vi "Read ZY_control.vi"(8 "error in (no error)":errorcluster, 11 "reg in":refnum<class "bronkhorst_reg_1.lvclass">) -> (0 "error out":errorcluster, 2 "ZY_control":T1={"Start"=FALSE, "Z_HSw"=0, "Z_HSetState"=enum."on", "Y_HSw"=0, "Y_HSetState"=enum."hand", "SP"=0.0, "Y_H"=0.0, "Reset_ALR"=FALSE} {"Y_H" step=1.0; "SP" step=0.01 format="%.2f"}, 3 "reg out":refnum<class "bronkhorst_reg_1.lvclass">)   [LabVIEW 2019, in "bronkhorst_reg_1.lvclass"]
uses:
  bronkhorst_reg_1.lvclass
  ctl/ZY_control_short.ctl
  ctl/Z_State.ctl
  ctl/Y_state.ctl
  bronkhorst_reg_1.lvclass/bronkhorst_reg_1.ctl
  control.lvlib
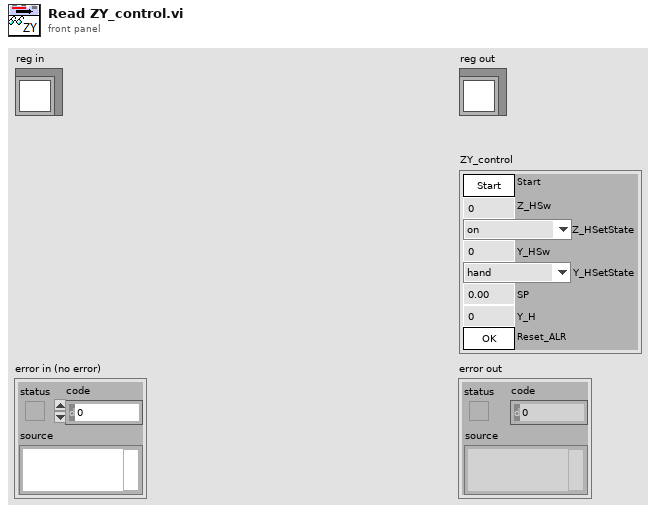
[diagram p1: front panel]
types:
  T1 = typedef "control.lvlib/ZY_control_short.ctl" = cluster{"Start":bool, "Z_HSw":u32, "Z_HSetState":T2, "Y_HSw":u32, "Y_HSetState":T3, "SP":dbl, "Y_H":dbl, "Reset_ALR":bool}
  T2 = typedef "control.lvlib/Z_State.ctl" = enum8{"initialization", "alarm", "disabled", "not ready", "stop ready", "reserv", "switched off", "reserv2", "switched on", "check", "on min", "decrease out", "on", "increase out", "on max"}
  T3 = typedef "control.lvlib/Y_state.ctl" = enum8{"initialize", "alarm", "min", "stop", "hand", "auto", "max"}
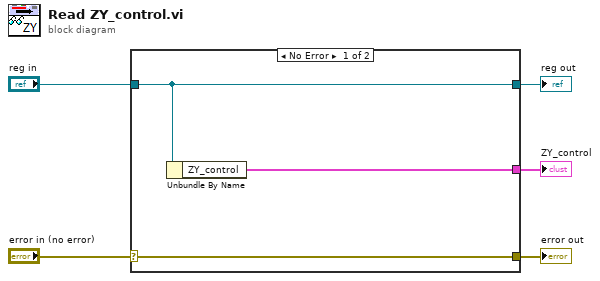
[diagram p0: block diagram]
diagram:
  n1 = case shown="No Error" "error in (no error)" {
    selector: "error in (no error)" -> [w8 w9]
    tunnel: [w8 w9] -> w4
    tunnel: [w7 w10] -> w2
    tunnel: "reg in" -> [w7 w10]
    tunnel: [w6 _] -> w1
    frame No Error {
      n2 = Unbundle By Name(w7) -> ("ZY_control"=w6:T1)
    }
    frame Error {
    }
  }
  "error out" <- w4
  "reg out" <- w2
  "ZY_control" <- w1
